vi "IOProcessPanel.vi"() -> ()   [LabVIEW 2019]
uses:
  LLB/Commonly VI/Main Glb.vi
  GLB/IO Process GLB.vi
  Class/Main Process Class/MPC_VirbVision/Panel RefGlb.vi
  LLB/Commonly VI.lvlib
panel:
  in  "Btn_RemoveAlgorithm":bool
  in  "Btn_Add Algorithm":bool
  in  "AlgParameter":string
  in  "Algorithm List":i32(listbox)
  in  "SubUI":bool=TRUE
  in  "Btn_Load":bool
  out "Root Path":path
  in  "DataTable":T1(array[cluster])
  in  "Enum_Algorithm":enum16{"CG_Histogram", "C_Color Matching"}(ring)
  in  "Tab Control":enum32{"Page 1"}(tab)
  in  "Tab Control 2":enum32{"OutPut", "Input", "Wait"}(tab)
  in  "OutStatus":bool caption="輸出狀態"
  in  "OutputPoint":u16(ring) caption="輸出點位" items=["Out_0", "Out_1", "Out_2", "Out_3", "Out_4", "Out_5", "Out_6", "Out_7", "Out_8", "Out_9", "Out_10", "Out_11", "Out_12", "Out_13", "Out_14", "Out_15"]
  in  "Wait Time":i32 caption="等待時間(0.1S)" min=0
  in  "Btn_DelProject":bool
  in  "Btn_AddProject":bool
  in  "Btn_Save":bool
  in  "ProjectSet":u16(ring) caption="設定資料"
  in  "OutPutList":i32(listbox) caption="輸出列表"
  in  "Btn_ResultAdd":bool
  in  "Btn_Result Remove":bool
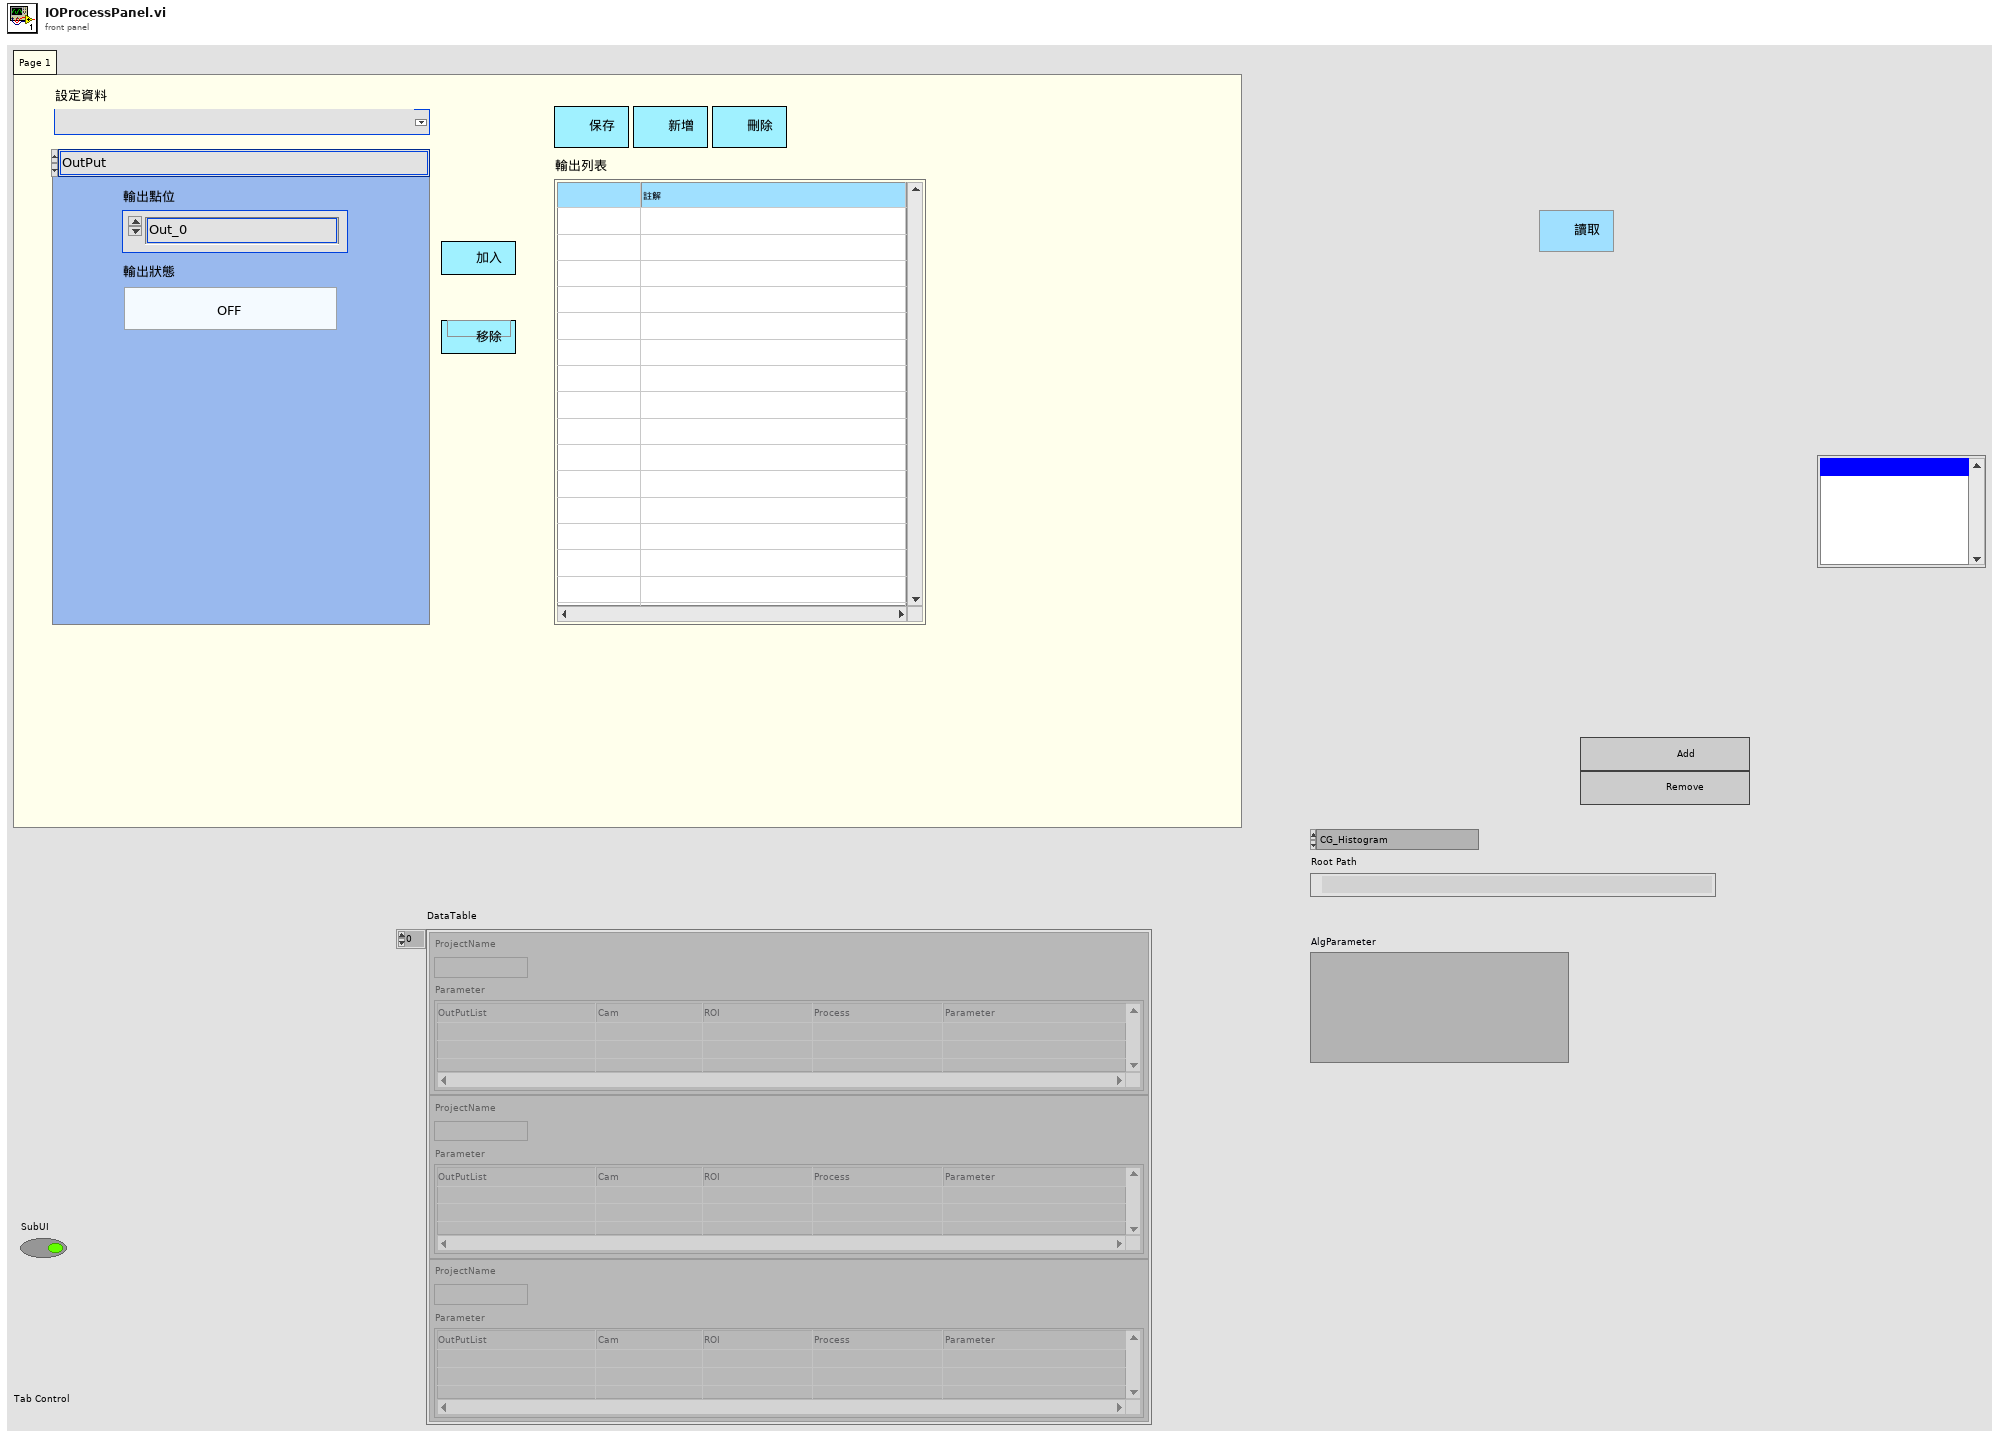
[diagram p1: front panel]
types:
  T1 = cluster{"ProjectName":string, "Parameter":string[][]}[]
  T2 = cluster{"ProjectName":string, "Parameter":string[][]}
  T3 = enum16{"initial", "write", "add", "delete", "Load", "Save", "Read", "ReadProjectName"}
  T4 = enum32{"invalid app kind", "Development System", "Run Time System", "Student Edition", "Embedded LabVIEW", "Evaluation", "Custom"}
  T5 = cluster{"RingText.Text":string, "ItemNames":string[][]}
  T6 = typedef "LVPoint32TypeDef.ctl" = cluster{"Horizontal":i32, "Vertical":i32}
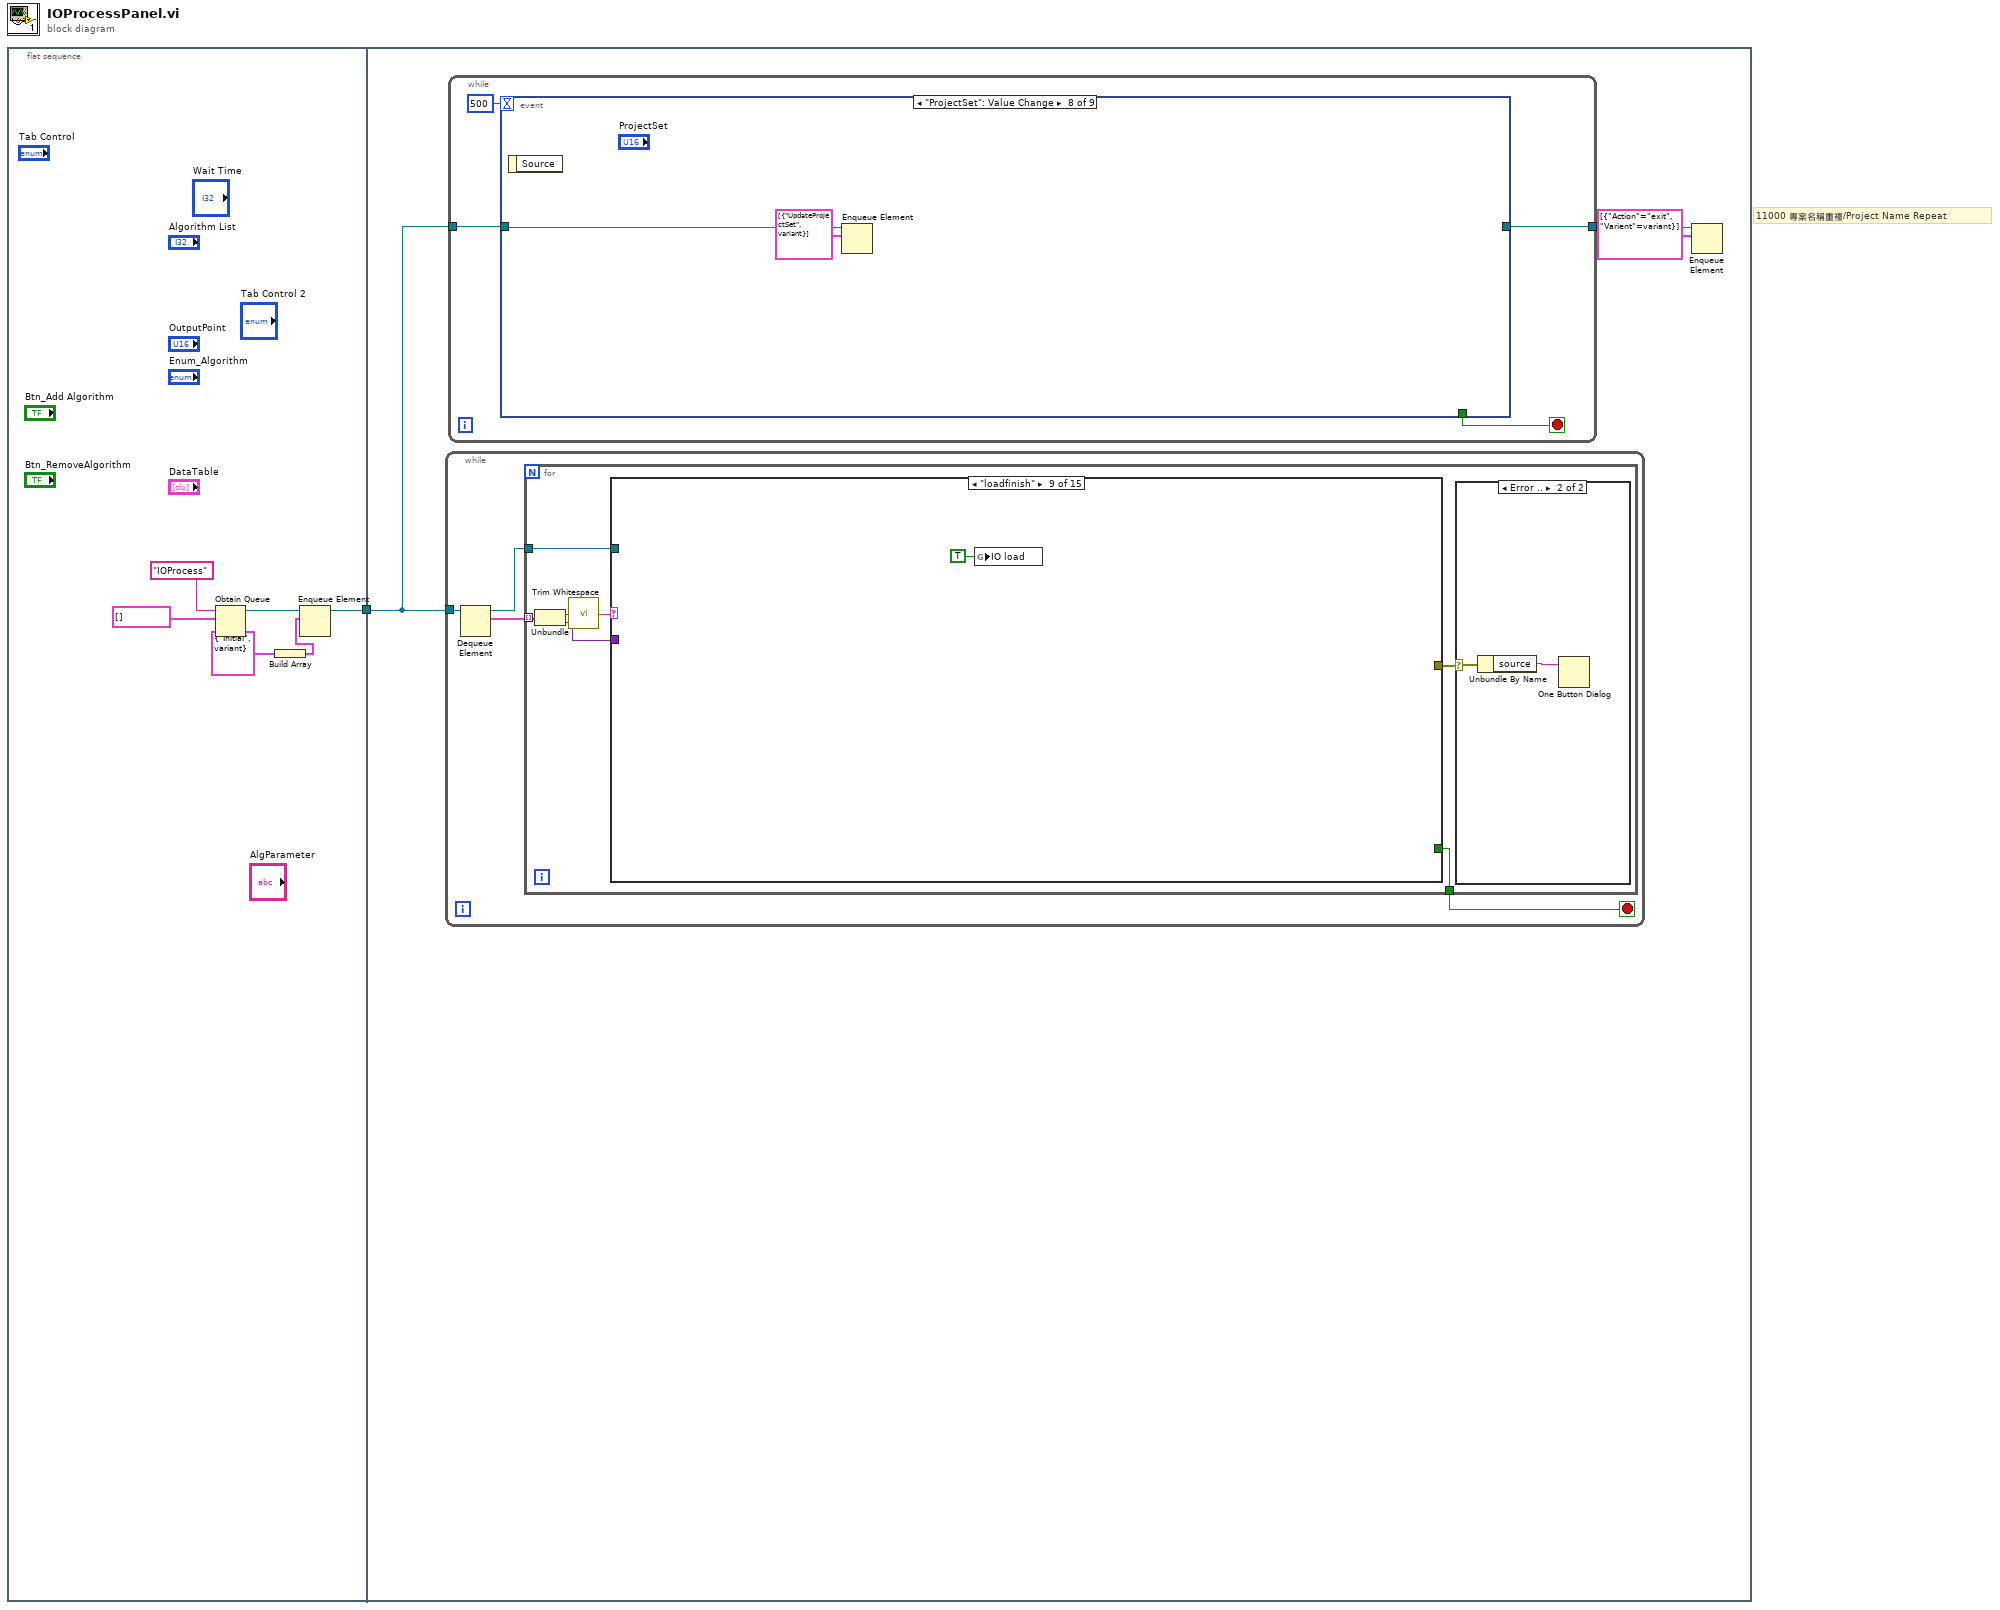
[diagram p0: block diagram]
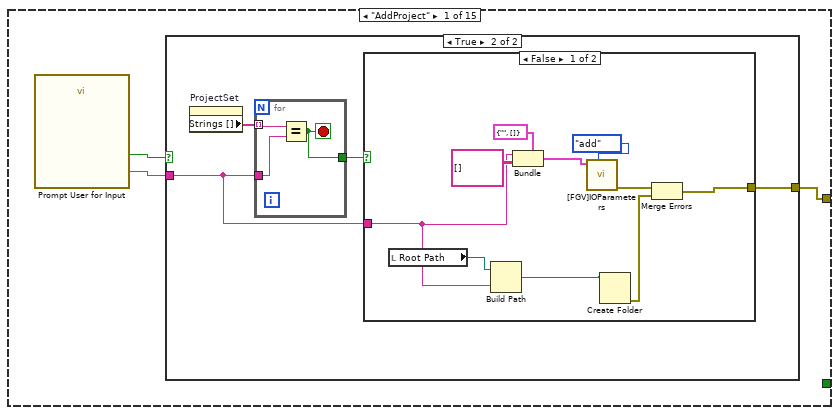
[diagram p3: hidden frame]
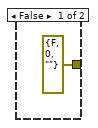
[diagram p4: hidden frame]
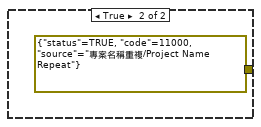
[diagram p5: hidden frame]
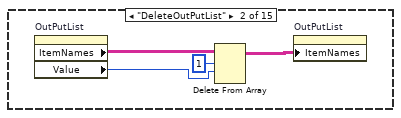
[diagram p6: hidden frame]
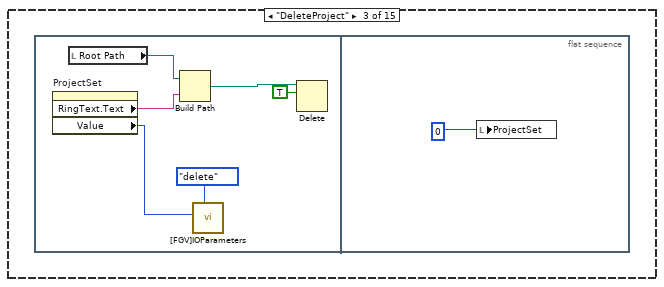
[diagram p7: hidden frame]
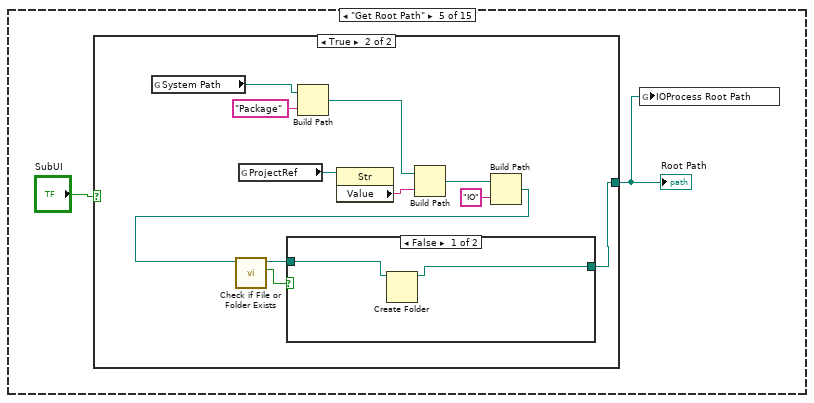
[diagram p9: hidden frame]
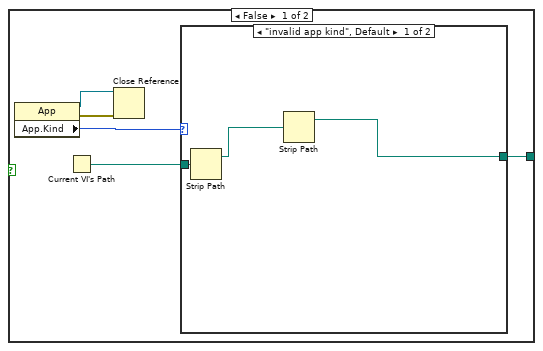
[diagram p10: hidden frame]
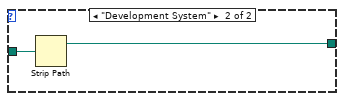
[diagram p11: hidden frame]
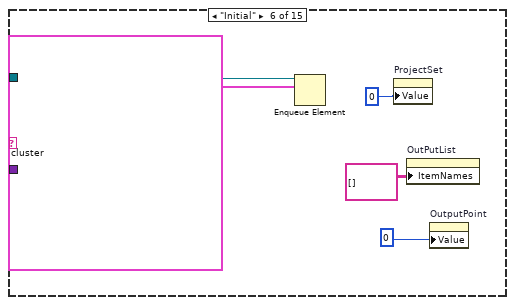
[diagram p13: hidden frame]
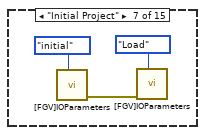
[diagram p14: hidden frame]
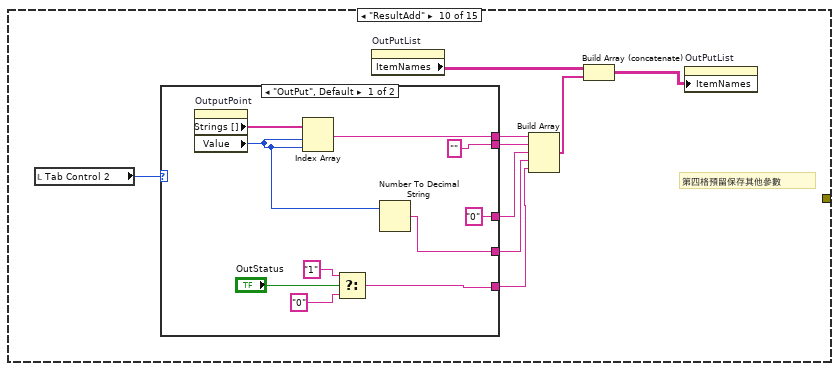
[diagram p16: hidden frame]
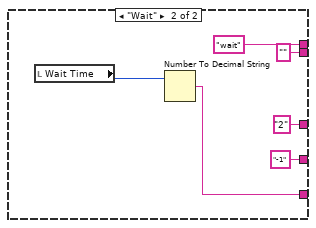
[diagram p17: hidden frame]
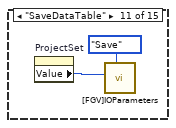
[diagram p18: hidden frame]
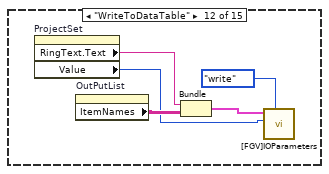
[diagram p19: hidden frame]
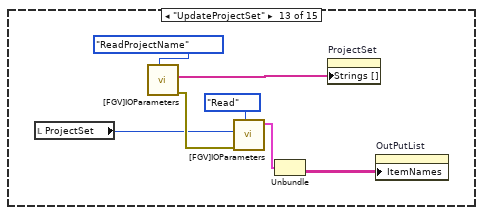
[diagram p20: hidden frame]
diagram:
  # "11000 專案名稱重複/Project Name Repeat"
  n1 = flat-sequence {
    tunnel: [w5] -> w1
    tunnel: w1 -> [w10]
    frame #0 {
      n2 = Obtain Queue(name (unnamed)="IOProcess", element data type=cluster{"Action":string, "Varient":variant}[] []) -> (queue out=w6:refnum<queue>)  [unwired: 3 in, 2 out]
      n3 = Build Array(cluster{"Action":string, "Varient":variant} {"Action"="Initial", "Varient"=variant} ("element")) -> (w2:cluster{"Action":string, "Varient":variant}[])
      n4 = Enqueue Element(queue=w6, element=w2) -> (queue out=w5:refnum<queue>)  [unwired: 2 in, 2 out]
    }
    frame #1 {
      n5 = while {
        tunnel: w10 -> [w14]
        stop <- w11 stop-if-true
        n6 = Dequeue Element(queue=w14) -> (queue out=w12:refnum<queue>, element=w13:cluster{"Action":string, "Varient":variant}[])  [unwired: 2 in, 2 out]
        n7 = for {
          tunnel: w13 -> [w21] mode=indexing
          tunnel: w12 -> [w19]
          tunnel: [w17] -> w11
          n8 = Unbundle(w21) -> ("Action"=w20:string, "Varient"=w15:variant)
          n9 = call <vilib>:"Trim Whitespace.vi"("string"=w20) -> ("trimmed string"=w16:string)  [unwired: 1 in]
          n10 = case shown="\"loadfinish\"" w16 {
            tunnel: w19 -> [_ _ _ _ _ w87 _ _ _ _ _ _ _ _ _]
            tunnel: [w24 _ _ _ _ _ _ _ _ _ _ _ _ _ _] -> w18
            tunnel: [_ _ _ _ _ _ _ _ _ _ _ _ _ _ w145] -> w17
            tunnel: w15 -> [_ _ _ _ _ _ _ _ _ _ _ _ _ _ _]
            frame "AddProject" {
              n11 = call "Prompt User for Input"() -> ("名稱/Name"=w26:string, "OK"=w25:bool)  [unwired: 17 in, 1 out]
              n12 = case shown="True" w25 {
                tunnel: w26 -> [_ w28]
                tunnel: [errorcluster {"status"=FALSE, "code"=0, "source"=""} ("error constant") w29] -> w24
                frame False {
                }
                frame True {
                  n13 = property on="ProjectSet" class="Ring (strict)"() -> ("Strings []"=w31:string[])  [unwired: 2 in, 2 out]
                  n14 = for {
                    tunnel: w31 -> [w45] mode=indexing
                    tunnel: w28 -> [w44]
                    tunnel: [w43] -> w30
                    stop <- w43 stop-if-true
                    n15 = Equal?(x=w45, y=w44) -> (x = y?=w43:bool)
                  }
                  n16 = case shown="False" w30 {
                    tunnel: [w33 errorcluster {"status"=TRUE, "code"=11000, "source"="專案名稱重複/Project Name Repeat"} ("error constant")] -> w29
                    tunnel: w28 -> [w36 _]
                    frame False {
                      n17 = local read "Root Path"() -> (w34:path)
                      n18 = Build Path(base path=w34, name or relative path=w36) -> (appended path=w35:path)
                      n19 = Bundle(cluster=T2 {"ProjectName"="", "Parameter"=[]} ("DataIn"), "ProjectName"=w36, "Parameter"=string[][] []) -> (w38:T2)
                      n20 = call "[FGV]IOParameters.vi"("Enum"=T3."add", "DataIn"=w38) -> ("error out"=w40:errorcluster)  [unwired: 7 in, 2 out]
                      n21 = Create Folder(path (use dialog)=w35) -> (error out=w32:errorcluster)  [unwired: 2 in, 2 out]
                      n22 = Merge Errors(w40, w32) -> (w33:errorcluster)
                    }
                    frame True {
                    }
                  }
                }
              }
            }
            frame "DeleteOutPutList" {
              n23 = property on="OutPutList" class="MCListbox (strict)"() -> ("ItemNames"=w49:string[][], "Value"=w47:i32)  [unwired: 2 in, 2 out]
              n24 = Delete From Array(array=w49, length=1, index (row)=w47) -> (array with subset deleted=w46:string[][])  [unwired: 1 in, 1 out]
              n25 = property on="OutPutList" class="MCListbox (strict)"("ItemNames"=w46) -> ()  [unwired: 2 in, 2 out]
            }
            frame "DeleteProject" {
              n26 = flat-sequence {
                frame #0 {
                  n27 = property on="ProjectSet" class="Ring (strict)"() -> ("RingText.Text"=w54:string, "Value"=w50:u16)  [unwired: 2 in, 2 out]
                  n28 = local read "Root Path"() -> (w55:path)
                  n29 = Build Path(base path=w55, name or relative path=w54) -> (appended path=w53:path)
                  n30 = call "[FGV]IOParameters.vi"("Enum"=T3."delete", "ProjectIndex"=w50) -> ()  [unwired: 7 in, 3 out]
                  n31 = Delete(path (use dialog)=w53, entire hierarchy (F)=TRUE) -> ()  [unwired: 3 in, 3 out]
                }
                frame #1 {
                  n32 = local write "ProjectSet"(0) -> ()
                }
              }
            }
            frame "False", Default {
            }
            frame "Get Root Path" {
              n33 = case shown="True" "SubUI" {
                tunnel: [w59 w70] -> w57
                frame False {
                  n34 = property class="App"() -> (reference out=w60:refnum<vi>, error out=w61:errorcluster, "App.Kind"=w63:T4)  [unwired: 2 in]
                  n35 = Current VI's Path() -> (path=w62:path)
                  n36 = Close Reference(reference=w60, error in (no error)=w61) -> ()  [unwired: 1 out]
                  n37 = case shown="\"invalid app kind\", Default" w63 {
                    tunnel: w62 -> [w66 w68]
                    tunnel: [w64 w67] -> w59
                    frame "invalid app kind", Default {
                      n38 = Strip Path(path=w66) -> (stripped path=w65:path)  [unwired: 1 out]
                      n39 = Strip Path(path=w65) -> (stripped path=w64:path)  [unwired: 1 out]
                    }
                    frame "Development System" {
                      n40 = Strip Path(path=w68) -> (stripped path=w67:path)  [unwired: 1 out]
                    }
                  }
                }
                frame True {
                  n41 = global read "Main Glb.vi" "System Path"() -> (w77:path)
                  n42 = global read "Main Glb.vi" "ProjectRef"() -> (w79:refnum<vi>)
                  n43 = Build Path(base path=w77, name or relative path="Package") -> (appended path=w76:path)
                  n44 = property class="Str"(reference=w79) -> ("Value"=w78:string)  [unwired: 1 in, 2 out]
                  n45 = Build Path(base path=w76, name or relative path=w78) -> (appended path=w74:path)
                  n46 = Build Path(base path=w74, name or relative path="IO") -> (appended path=w72:path)
                  n47 = call <vilib>:"Check if File or Folder Exists.vi"("path"=w72) -> ("file or folder exists?"=w71:bool, "dup path"=w69:path)  [unwired: 8 in, 1 out]
                  n48 = case shown="False" w71 {
                    tunnel: [w80 w82] -> w70
                    tunnel: w69 -> [w81 w82]
                    frame False {
                      n49 = Create Folder(path (use dialog)=w81) -> (created path=w80:path)  [unwired: 2 in, 2 out]
                    }
                    frame True {
                    }
                  }
                }
              }
              "Root Path" <- w57
              n50 = global write "IO Process GLB.vi" "IOProcess Root Path"(w57) -> ()
            }
            frame "Initial" {
              n51 = Enqueue Element(queue=w87, element=cluster{"Action":string, "Varient":variant}[] [{"Action"="Get Root Path", "Varient"=variant}, {"Action"="Initial Project", "Varient"=variant}, {"Action"="UpdateProjectSet", "Varient"=variant}, {"Action"="Initial IOName", "Varient"=variant}]) -> ()  [unwired: 2 in, 3 out]
              n52 = property on="ProjectSet" class="Ring (strict)"("Value"=0) -> ()  [unwired: 2 in, 2 out]
              n53 = property on="OutPutList" class="MCListbox (strict)"("ItemNames"=string[][] [] ("Item Names")) -> ()  [unwired: 2 in, 2 out]
              n54 = property on="OutputPoint" class="Ring (strict)"("Value"=0) -> ()  [unwired: 2 in, 2 out]
            }
            frame "Initial Project" {
              n55 = call "[FGV]IOParameters.vi"("Enum"=T3."initial") -> ("error out"=w88:errorcluster)  [unwired: 8 in, 2 out]
              n56 = call "[FGV]IOParameters.vi"("Enum"=T3."Load", "error in"=w88) -> ()  [unwired: 7 in, 3 out]
            }
            frame "Initial IOName" {
            }
            frame "loadfinish" {
              n57 = global write "Panel RefGlb.vi" "IO load"(TRUE ("IO load")) -> ()
            }
            frame "ResultAdd" {
              # "第四格預留保存其他參數"
              n58 = local read "Tab Control 2"() -> (w96:enum32{"OutPut", "Input", "Wait"})
              n59 = case shown="\"OutPut\", Default" w96 {
                tunnel: ["0" "2"] -> w93
                tunnel: [w107 "wait"] -> w97
                tunnel: ["" ""] -> w94
                tunnel: [w102 "-1"] -> w95
                tunnel: [w101 w111] -> w92
                frame "OutPut", Default {
                  n60 = property on="OutputPoint" class="Ring (strict)"() -> ("Strings []"=w110:string[], "Value"=w109:u16)  [unwired: 2 in, 2 out]
                  n61 = Index Array(array=w110, index #1=w109, index #2=w109) -> (element #1=w107:string)  [unwired: 1 out]
                  n62 = Select(t="1", s="OutStatus", f="0") -> (s? t:f=w101:string)
                  n63 = Number To Decimal String(number=w109) -> (decimal integer string=w102:string)  [unwired: 1 in]
                }
                frame "Wait" {
                  n64 = local read "Wait Time"() -> (w116:i32)
                  n65 = Number To Decimal String(number=w116) -> (decimal integer string=w111:string)  [unwired: 1 in]
                }
              }
              n66 = property on="OutPutList" class="MCListbox (strict)"() -> ("ItemNames"=w100:string[][])  [unwired: 2 in, 2 out]
              n67 = Build Array(w97, w94, w93, w95, w92) -> (w99:string[])
              n68 = Build Array (concatenate)(w100, w99) -> (w98:string[][])
              n69 = property on="OutPutList" class="MCListbox (strict)"("ItemNames"=w98) -> ()  [unwired: 2 in, 2 out]
            }
            frame "SaveDataTable" {
              n70 = property on="ProjectSet" class="Ring (strict)"() -> ("Value"=w117:u16)  [unwired: 2 in, 2 out]
              n71 = call "[FGV]IOParameters.vi"("Enum"=T3."Save", "ProjectIndex"=w117) -> ()  [unwired: 7 in, 3 out]
            }
            frame "WriteToDataTable" {
              n72 = property on="ProjectSet" class="Ring (strict)"() -> ("RingText.Text"=w120:string, "Value"=w119:u16)  [unwired: 2 in, 2 out]
              n73 = property on="OutPutList" class="MCListbox (strict)"() -> ("ItemNames"=w122:string[][])  [unwired: 2 in, 2 out]
              n74 = Bundle("RingText.Text"=w120, "ItemNames"=w122) -> (w121:T5)  [unwired: 1 in]
              n75 = call "[FGV]IOParameters.vi"("Enum"=T3."write", "ProjectIndex"=w119, "DataIn"=w121) -> ()  [unwired: 6 in, 3 out]
            }
            frame "UpdateProjectSet" {
              n76 = local read "ProjectSet"() -> (w124:u16)
              n77 = call "[FGV]IOParameters.vi"("Enum"=T3."ReadProjectName") -> ("error out"=w128:errorcluster, "ProjectName"=w130:string[])  [unwired: 8 in, 1 out]
              n78 = call "[FGV]IOParameters.vi"("Enum"=T3."Read", "error in"=w128, "ProjectIndex"=w124) -> ("DataOut"=w126:T2)  [unwired: 6 in, 2 out]
              n79 = Unbundle(w126) -> ("Parameter"=w125:string[][])  [unwired: 1 out]
              n80 = property on="ProjectSet" class="Ring (strict)"("Strings []"=w130) -> ()  [unwired: 2 in, 2 out]
              n81 = property on="OutPutList" class="MCListbox (strict)"("ItemNames"=w125) -> ()  [unwired: 2 in, 2 out]
            }
            frame "UpDataSetPanel" {
              # "IOName,Describe,Type,IOIndex,Data"
              n82 = property on="OutPutList" class="MCListbox (strict)"() -> ("ItemNames"=w138:string[][], "Value"=w137:i32)  [unwired: 2 in, 2 out]
              n83 = Index Array(array=w138, index (row)=w137) -> (element=w136:string[])  [unwired: 1 in]
              n84 = Index Array(array=w136) -> (element #3=w135:string, element #4=w133:string, element #5=w131:string)  [unwired: 5 in, 2 out]
              n85 = Decimal String To Number(string=w133) -> (number=w132:i32)  [unwired: 2 in, 1 out]
              n86 = Decimal String To Number(string=w135) -> (number=w134:i32)  [unwired: 2 in, 1 out]
              n87 = case shown="0, Default" w134 {
                tunnel: w132 -> [w142 _ _]
                tunnel: w131 -> [w141 _ w144]
                frame 0, Default {
                  n88 = local write "OutputPoint"(w142) -> ()
                  n89 = Equal?(x=w141, y="1") -> (x = y?=w139:bool)
                  n90 = local write "OutStatus"(w139) -> ()
                }
                frame 1 {
                }
                frame 2 {
                  n91 = Decimal String To Number(string=w144) -> (number=w143:i32)  [unwired: 2 in, 1 out]
                  n92 = local write "Wait Time"(w143) -> ()
                }
              }
              n93 = local write "Tab Control 2"(w134) -> ()
            }
            frame "exit" {
              n94 = call "Exit.vi"("Enum"=enum16{"Initial", "Read", "Write"}."Read") -> ("ExitOut"=w145:bool)  [unwired: 10 in]
            }
          }
          n95 = case shown="Error .." w18 {
            selector: w18 -> [_ w23]
            frame No Error {
            }
            frame Error {
              n96 = Unbundle By Name(w23) -> ("source"=w22:string)
              n97 = One Button Dialog(message=w22) -> ()  [unwired: 1 in, 1 out]
            }
          }
        }
      }
      n98 = while {
        tunnel: w10 -> [w148]
        tunnel: [w147] -> w9
        stop <- w150 stop-if-true
        n99 = event shown="[7] \"ProjectSet\": Value Change" {
          selector: _ -> [_ _ _ _ _ _ _ _ _]
          dyn-events: _ -> [_ _ _ _ _ _ _ _ _]
          timeout: 500 -> [_ _ _ _ _ _ _ _ _]
          tunnel: [_ _ _ _ _ _ _ _ w191] -> w150
          tunnel: w148 -> [w152 w153 w161 w163 w164 w175 w179 w188 w189]
          tunnel: [_ _ _ _ _ _ _ _ w189] -> w147
          event "Btn_AddProject": Value Change {
            n100 = event-data() -> ()  [unwired: 1 in, 1 out]
            n101 = Enqueue Element(queue=w152, element=cluster{"Action":string, "Varient":variant}[] [{"Action"="AddProject", "Varient"=variant}, {"Action"="UpdateProjectSet", "Varient"=variant}]) -> ()  [unwired: 2 in, 3 out]
          }
          event "Btn_DelProject": Value Change {
            n102 = event-data() -> ()  [unwired: 1 in, 2 out]
            n103 = property on="ProjectSet" class="Ring (strict)"() -> ("RingText.Text"=w156:string)  [unwired: 2 in, 2 out]
            n104 = Format Into String(format string="確認是否刪除專案:%s\nCheck Delete Project : %s", w156, w156) -> (resulting string=w155:string)  [unwired: 2 in, 1 out]
            n105 = Two Button Dialog(message=w155) -> (T button?=w154:bool)  [unwired: 2 in]
            n106 = case shown="True" w154 {
              tunnel: w153 -> [_ w159]
              frame False {
              }
              frame True {
                n107 = Enqueue Element(queue=w159, element=cluster{"Action":string, "Varient":variant}[] [{"Action"="DeleteProject", "Varient"=variant}, {"Action"="UpdateProjectSet", "Varient"=variant}]) -> ()  [unwired: 2 in, 3 out]
              }
            }
          }
          event "Btn_Load": Value Change {
            n108 = event-data() -> ()  [unwired: 1 in, 1 out]
            n109 = Enqueue Element(queue=w161, element=cluster{"Action":string, "Varient":variant}[] [{"Action"="UpDateDataToUI", "Varient"=variant}]) -> ()  [unwired: 2 in, 3 out]
          }
          event "Btn_ResultAdd": Value Change {
            n110 = event-data() -> ()  [unwired: 1 in, 1 out]
            n111 = Enqueue Element(queue=w163, element=cluster{"Action":string, "Varient":variant}[] [{"Action"="ResultAdd", "Varient"=variant}]) -> ()  [unwired: 2 in, 3 out]
          }
          event "Btn_Result Remove": Value Change {
            n112 = event-data() -> ()  [unwired: 1 in, 1 out]
            n113 = property on="OutPutList" class="MCListbox (strict)"() -> ("ItemNames"=w171:string[][], "Value"=w170:i32)  [unwired: 2 in, 2 out]
            n114 = Index Array(array=w171, index (row)=w170, index (col)=0 ("disabled index (col)")) -> (element=w167:string)
            n115 = Format Into String(format string="確認是否刪除輸出資料%s?\nMake Sure Delete Output Parameter %s?", w167, w167) -> (resulting string=w166:string)  [unwired: 2 in, 1 out]
            n116 = Two Button Dialog(message=w166) -> (T button?=w165:bool)  [unwired: 2 in]
            n117 = case shown="True" w165 {
              tunnel: w164 -> [_ w173]
              frame False {
              }
              frame True {
                n118 = Enqueue Element(queue=w173, element=cluster{"Action":string, "Varient":variant}[] [{"Action"="DeleteOutPutList", "Varient"=variant}]) -> ()  [unwired: 2 in, 3 out]
              }
            }
          }
          event "Btn_Save": Value Change {
            n119 = event-data() -> ()  [unwired: 1 in, 2 out]
            n120 = Enqueue Element(queue=w175, element=cluster{"Action":string, "Varient":variant}[] [{"Action"="WriteToDataTable", "Varient"=variant}, {"Action"="SaveDataTable", "Varient"=variant}]) -> ()  [unwired: 2 in, 3 out]
          }
          event "OutPutList": Mouse Down {
            n121 = event-data() -> ("Mods.Double Click"=w178:bool, "Coords"=w177:T6)  [unwired: 1 in, 1 out]
            n122 = case shown="True" w178 {
              tunnel: w179 -> [w181 w185]
              tunnel: w177 -> [_ w183]
              tunnel: "OutPutList" -> [_ w182]
              frame False {
                n123 = Enqueue Element(queue=w181, element=cluster{"Action":string, "Varient":variant}[] [{"Action"="UpDataSetPanel", "Varient"=variant}]) -> ()  [unwired: 2 in, 3 out]
              }
              frame True {
                n124 = control-ref of="OutPutList"() -> (w184:refnum<vi>)
                n125 = call "List Mousedown Edit.vi"("Row"=w182, "Coords"=w183, "Listbox in"=w184) -> ()  [unwired: 9 in]
                n126 = Enqueue Element(queue=w185, element=cluster{"Action":string, "Varient":variant}[] [{"Action"="UpDataSetPanel", "Varient"=variant}]) -> ()  [unwired: 2 in, 3 out]
              }
            }
          }
          event "ProjectSet": Value Change {
            n127 = event-data() -> ()  [unwired: 1 in, 1 out]
            n128 = Enqueue Element(queue=w188, element=cluster{"Action":string, "Varient":variant}[] [{"Action"="UpdateProjectSet", "Varient"=variant}]) -> ()  [unwired: 2 in, 3 out]
          }
          event Timeout {
            n129 = event-data() -> ()  [unwired: 1 in, 3 out]
            n130 = call "Exit.vi"("Enum"=enum16{"Initial", "Read", "Write"}."Read") -> ("ExitOut"=w191:bool)  [unwired: 10 in]
          }
        }
      }
      n131 = Enqueue Element(queue=w9, element=cluster{"Action":string, "Varient":variant}[] [{"Action"="exit", "Varient"=variant}]) -> ()  [unwired: 2 in, 3 out]
    }
  }
